vi "ExtRefSource_set.vi"(10 "extrefs/0/enable":T2) -> (2 "zi_node":T1)   [LabVIEW 2016]
uses:
  Controls/ExtRefSource.ctl
  Controls/zi_node.ctl
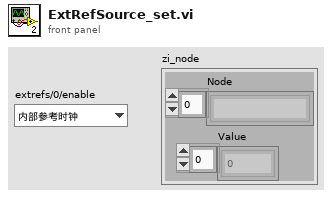
[diagram p1: front panel]
types:
  T1 = typedef "zi_node.ctl" = cluster{"Node":string[], "Value":dbl[]}
  T2 = typedef "ExtRefSource.ctl" = enum16{"内部参考时钟", "外部参考时钟/Aux Input 1", "外部参考时钟/Trigger 1"}
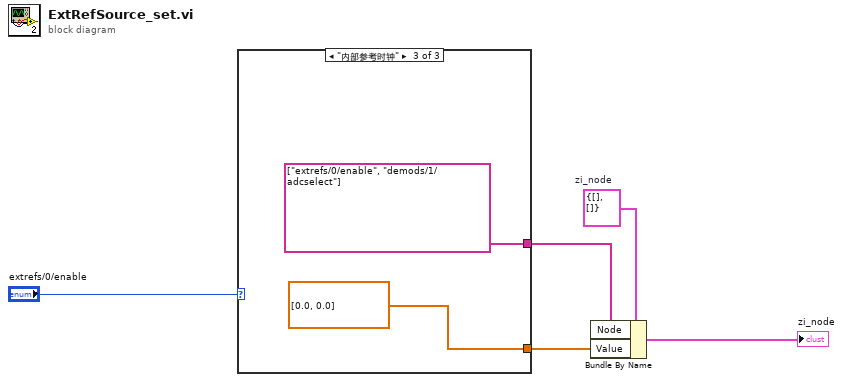
[diagram p0: block diagram]
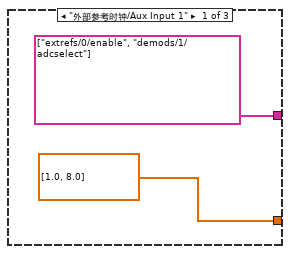
[diagram p2: hidden frame]
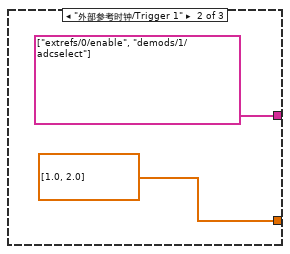
[diagram p3: hidden frame]
diagram:
  w1 = T1 {"Node"=[], "Value"=[]}  # zi_node
  n1 = case shown="\"内部参考时钟\"" "extrefs/0/enable" {
    tunnel: [string[] ["extrefs/0/enable", "demods/1/adcselect"] string[] ["extrefs/0/enable", "demods/1/adcselect"] string[] ["extrefs/0/enable", "demods/1/adcselect"]] -> w4
    tunnel: [dbl[] [1.0, 8.0] dbl[] [1.0, 2.0] dbl[] [0.0, 0.0]] -> w5
    frame "外部参考时钟/Aux Input 1" {
    }
    frame "外部参考时钟/Trigger 1" {
    }
    frame "内部参考时钟" {
    }
  }
  n2 = Bundle By Name(cluster=w1, "Node"=w4, "Value"=w5) -> (→"zi_node":T1)
